vi "Init.vi"(0 "SystemEvents in":refnum<class "SystemEvents.lvclass">, 1 "Events":T1, 5 "error in (no error)":errorcluster) -> (14 "SystemEvents out":refnum<class "SystemEvents.lvclass">, 19 "error out":errorcluster)   [LabVIEW 2017, in "SystemEvents.lvclass"]
doc: "Creates user events for all events in the 'Events' cluster and stores these in the object attributes."
uses:
  SystemEvents.lvclass
  SystemEventData/SystemEventsType.ctl
  SystemEvents.lvclass/SystemEvents.ctl
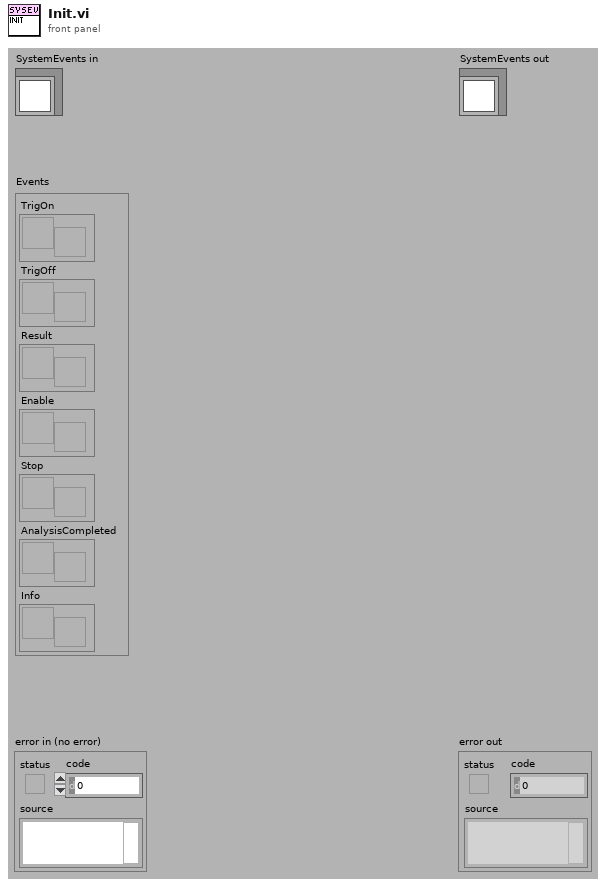
[diagram p1: front panel]
types:
  T1 = typedef "SystemEventsType.ctl" = cluster{"TrigOn":refnum<user-event>, "TrigOff":refnum<user-event>, "Result":refnum<user-event>, "Enable":refnum<user-event>, "Stop":refnum<user-event>, "AnalysisCompleted":refnum<user-event>, "Info":refnum<user-event>}
  T2 = cluster{"[0]":refnum<user-event>, "[1]":refnum<user-event>, "[2]":refnum<user-event>, "[3]":refnum<user-event>, "[4]":refnum<user-event>, "[5]":refnum<user-event>, "[6]":refnum<user-event>}
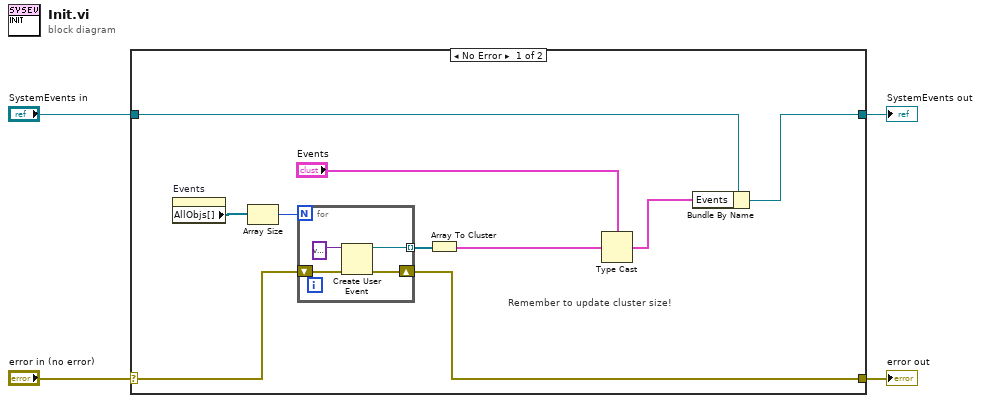
[diagram p0: block diagram]
diagram:
  n1 = case shown="No Error" "error in (no error)" {
    selector: "error in (no error)" -> [w6 w20]
    tunnel: [w5 w20] -> w3
    tunnel: [w13 w19] -> w1
    tunnel: "SystemEvents in" -> [w14 w19]
    frame No Error {
      # "Remember to update cluster size!"
      n2 = property on="Events" class="Clust (strict)"() -> ("AllObjs[]"=w12:refnum<vi>[])  [unwired: 2 in, 2 out]
      n3 = Array Size(array=w12) -> (size(s)=w11:i32)
      n4 = for {
        N: w11 -> [_]
        shift-right: [w16] -> w5
        shift-left: w6 -> [w17]
        tunnel: [w15] -> w10 mode=indexing
        n5 = Create User Event(user event datatype=variant ("variant"), error in=w17) -> (user event=w15:refnum<user-event>, error out=w16:errorcluster)
      }
      n6 = Array To Cluster(array=w10) -> (cluster=w9:T2)
      n7 = Type Cast(type="Events", x=w9) -> (*(type *) &x=w7:T1)
      n8 = Bundle By Name(cluster=w14, "Events"=w7) -> (w13:refnum<class "SystemEvents.lvclass">)
    }
    frame Error {
    }
  }
  "error out" <- w3
  "SystemEvents out" <- w1
